vi "Create Framework Status.vi"(8 "error in (no error)":errorcluster, 11 "Framework Configuration":T1) -> (0 "error out":errorcluster, 3 "Framework Status":refnum<class "Framework Status.lvclass">)   [LabVIEW 2017, in "DSF Core.lvlib" / "Framework Status.lvclass"]
uses:
  Framework Status.lvclass
  Typedefs/DSF Engine Framework Configuration.ctl
  Typedefs/DSF Engine Plugin Configuration.ctl
  Typedefs/DSF Timing Info.ctl
  Typedefs/DSF Engine Plugin Thread Configuration.ctl
  Typedefs/DSF Settings Info.ctl
  Typedefs/DSF Engine Transfer Group Configuration.ctl
  Typedefs/DSF Direction.ctl
  Typedefs/DSF Engine Transfer Configuration.ctl
  Typedefs/DSF Byte Order.ctl
  Typedefs/DSF Engine Channel Configuration.ctl
  Typedefs/DSF Data Type.ctl
  Typedefs/DSF Timeout Behavior.ctl
  Framework Status.lvclass/Framework Status.ctl
  Configuration/Transfer Group Count (Framework).vi
  Transfer Group Status/Status.lvclass
  DSF Core.lvlib
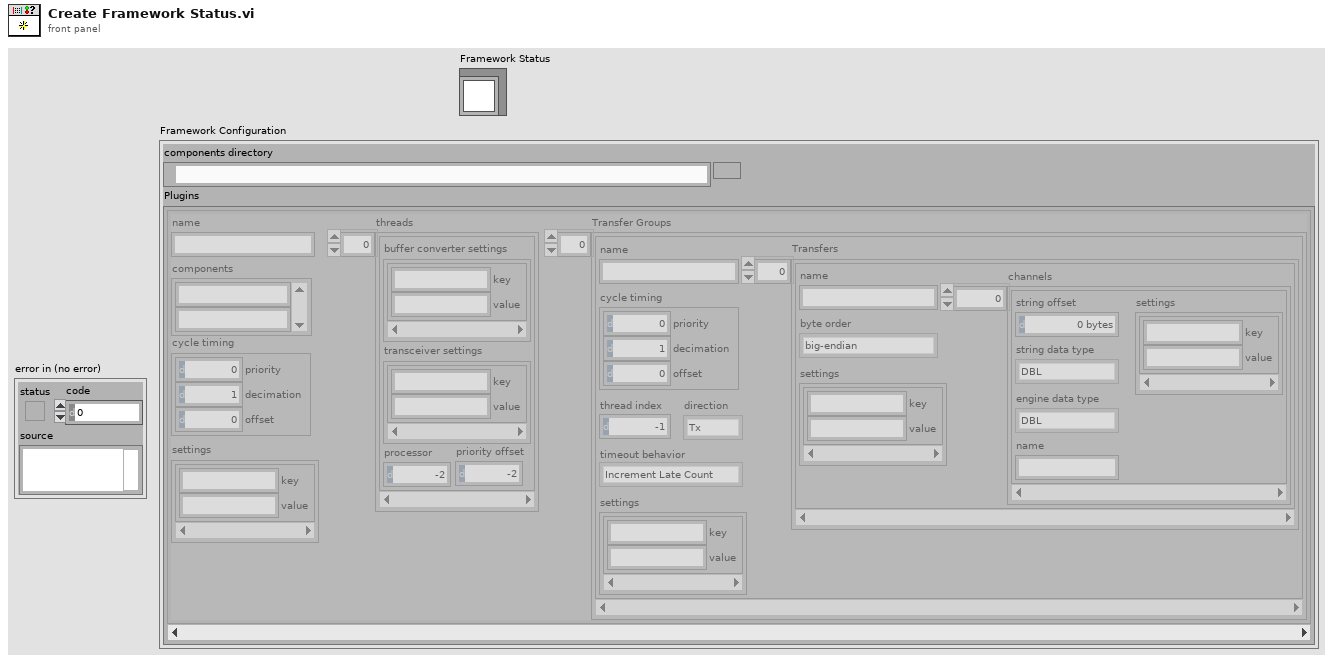
[diagram p1: front panel]
types:
  T1 = typedef "DSF Core.lvlib/DSF Engine Framework Configuration.ctl" = cluster{"components directory":path, "Plugins":T2[]}
  T2 = typedef "DSF Core.lvlib/DSF Engine Plugin Configuration.ctl" = cluster{"name":string, "components":string[], "cycle timing":T3, "threads":T4[], "Transfer Groups":T6[], "settings":T5}
  T3 = typedef "DSF Core.lvlib/DSF Timing Info.ctl" = cluster{"priority":u64, "decimation":u64, "offset":u64}
  T4 = typedef "DSF Core.lvlib/DSF Engine Plugin Thread Configuration.ctl" = cluster{"buffer converter settings":T5, "transceiver settings":T5, "processor":i32, "priority offset":i16}
  T5 = typedef "DSF Core.lvlib/DSF Settings Info.ctl" = cluster{"key":string, "value":string}[]
  T6 = typedef "DSF Core.lvlib/DSF Engine Transfer Group Configuration.ctl" = cluster{"name":string, "direction":T7, "cycle timing":T3, "thread index":i32, "settings":T5, "Transfers":T8[], "timeout behavior":T12}
  T7 = typedef "DSF Core.lvlib/DSF Direction.ctl" = enum8{"Tx", "Rx"}
  T8 = typedef "DSF Core.lvlib/DSF Engine Transfer Configuration.ctl" = cluster{"name":string, "byte order":T9, "settings":T5, "channels":T10[]}
  T9 = typedef "DSF Core.lvlib/DSF Byte Order.ctl" = enum8{"big-endian", "little-endian"}
  T10 = typedef "DSF Core.lvlib/DSF Engine Channel Configuration.ctl" = cluster{"string offset":u64, "string data type":T11, "engine data type":T11, "name":string, "settings":T5}
  T11 = typedef "DSF Core.lvlib/DSF Data Type.ctl" = enum8{"Bool", "SGL", "DBL", "I8", "I16", "I32", "I64", "U8", "U16", "U32", "U64"}
  T12 = typedef "DSF Core.lvlib/DSF Timeout Behavior.ctl" = enum8{"Increment Late Count", "Throw Error"}
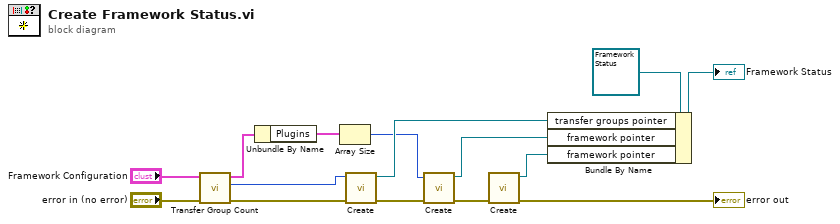
[diagram p0: block diagram]
diagram:
  n1 = call-poly "Transfer Group Count.vi"("error in (no error)"="error in (no error)", "Framework Configuration in"="Framework Configuration") -> ("error out"=w11:errorcluster, "transfer group count"=w12:i32, "Framework Configuration out"=w7:T1)  [unwired: 7 in]
  n2 = Unbundle By Name(w7) -> ("Plugins"=w6:T2[])
  n3 = Array Size(array=w6) -> (size(s)=w1:i32)
  n4 = call "Create.vi"("error in (no error)"=w11, "count (1)"=w12) -> ("error out"=w4:errorcluster, "status pointer"=w10:refnum<class "Status.lvclass">)  [unwired: 8 in]
  n5 = call "Create.vi"("error in (no error)"=w4, "count (1)"=w1) -> ("error out"=w3:errorcluster, "status pointer"=w2:refnum<class "Status.lvclass">)  [unwired: 8 in]
  n6 = call "Create.vi"("error in (no error)"=w3) -> ("error out"=→"error out":errorcluster, "status pointer"=w5:refnum<class "Status.lvclass">)  [unwired: 9 in]
  n7 = Bundle By Name(cluster=refnum<class "Framework Status.lvclass"> refnum ("Framework Status in"), "transfer groups pointer"=w10, "framework pointer"=w2, "framework pointer"=w5) -> (→"Framework Status":refnum<class "Framework Status.lvclass">)
